vi "Run All Unit Tests.vi"() -> ()   [LabVIEW 2016]
uses:
  <vilib>/addons/_JKI Toolkits/VI Tester/VI Tester API.llb/Run Tests (Path).vi
  <vilib>/addons/_JKI Toolkits/VI Tester/VI Tester API.llb/VI Tester API.lvlib
panel:
  out "test details":string
  out "successful?":bool
  in  "Test Path":path
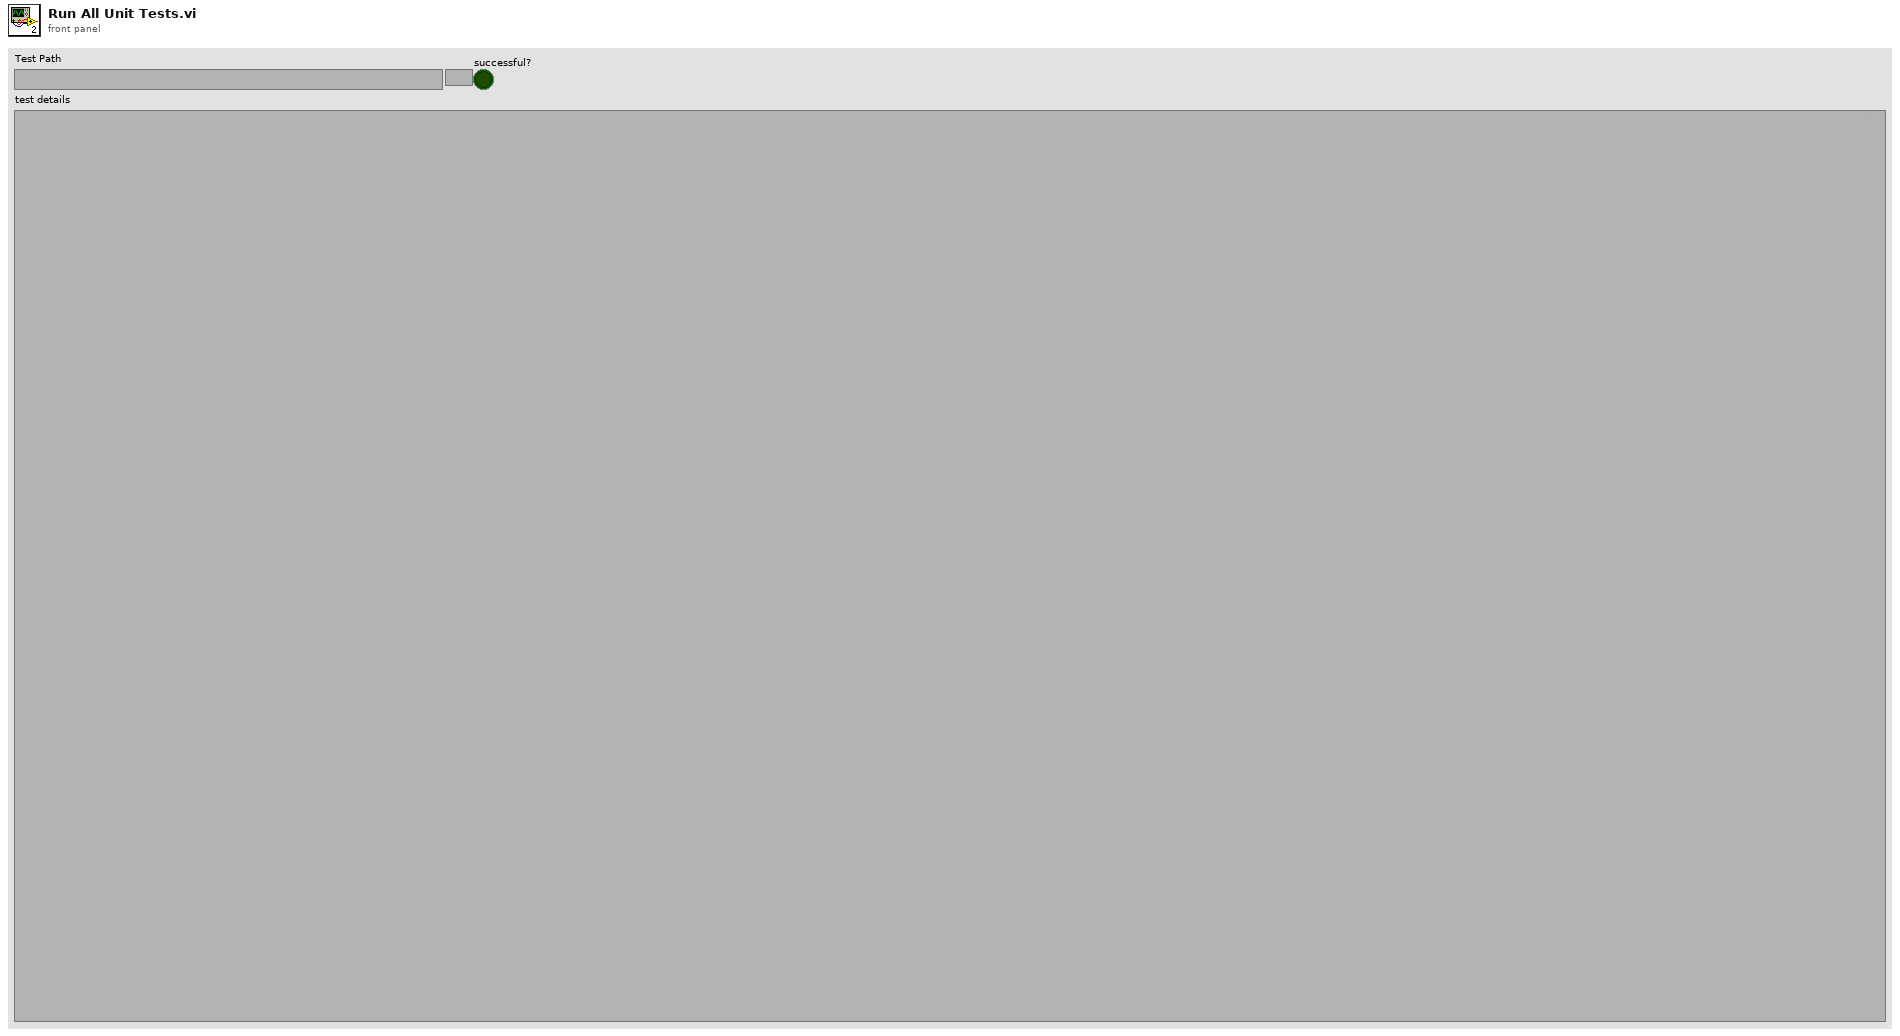
[diagram p1: front panel]
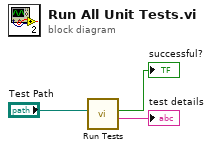
[diagram p0: block diagram]
diagram:
  n1 = call-poly <vilib>:"Run Tests.vi"("Test Path"="Test Path") -> ("test details"=→"test details":string, "successful?"=→"successful?":bool)  [unwired: 8 in, 1 out]
